vi "Verify Acquisition.vi"(8 "error in (no error)":errorcluster, 11 "CCDCamera in":refnum<class "Real Camera.lvclass">) -> (0 "error out":errorcluster, 3 "CCDCamera out":refnum<class "Real Camera.lvclass">)   [LabVIEW 2018, in "Real Camera.lvclass"]
doc: "Verify acquisition\n\nIf the camera is acquiring, the CCD status will be ACTIVE. Otherwise, it will be IDLE."
uses:
  Real Camera.lvclass
  C:/Users/Denis/Desktop/S4CCS/S4CCS/Simulated_CCD_Camera/Simulated Camera.lvclass
  Simulated_CCD_Camera/Simulated Camera.lvclass
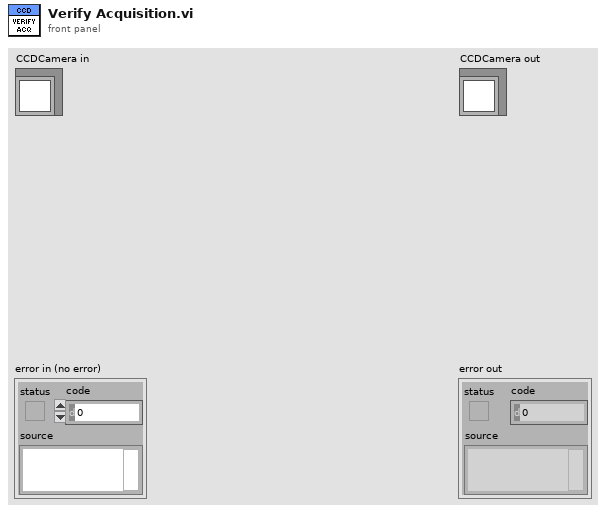
[diagram p1: front panel]
types:
  T1 = typedef "Error Code Enum typedef.ctl" = enum32{"N/A (0)", "DRV_ERROR_CODES", "DRV_SUCCESS", "DRV_VXDNOTINSTALLED", "DRV_ERROR_SCAN", "DRV_ERROR_CHECK_SUM", "DRV_ERROR_FILELOAD", "DRV_UNKNOWN_FUNC", "DRV_ERROR_VXD_INIT", "DRV_ERROR_ADDRESS", "DRV_ERROR_PAGELOCK", "DRV_ERROR_PAGEUNLOCK", "DRV_ERROR_BOARDTEST", "DRV_ERROR_ACK", "DRV_ERROR_UP_FIFO", "DRV_ERROR_PATTERN", "N/A (16)", "DRV_ACQUISITION_ERRORS", "DRV_ACQ_BUFFER", "DRV_ACQ_DOWNFIFO_FULL", "DRV_PROC_UNKONWN_INSTRUCTION", "DRV_ILLEGAL_OP_CODE", "DRV_KINETIC_TIME_NOT_MET", "DRV_ACCUM_TIME_NOT_MET", "DRV_NO_NEW_DATA", "N/A (25)", "DRV_SPOOLERROR", "N/A (27)", "N/A (28)", "N/A (29)", "N/A (30)", "N/A (31)", "N/A (32)", "DRV_TEMPERATURE_CODES", "DRV_TEMPERATURE_OFF", "DRV_TEMPERATURE_NOT_STABILIZED", "DRV_TEMPERATURE_STABILIZED", "DRV_TEMPERATURE_NOT_REACHED", "DRV_TEMPERATURE_OUT_RANGE", "DRV_TEMPERATURE_NOT_SUPPORTED", "DRV_TEMPERATURE_DRIFT", "N/A (41)", "N/A (42)", "N/A (43)", "N/A (44)", "N/A (45)", "N/A (46)", "N/A (47)", "N/A (48)", "DRV_GENERAL_ERRORS", "DRV_INVALID_AUX", "DRV_COF_NOTLOADED", "DRV_FPGAPROG", "DRV_FLEXERROR", "DRV_GPIBERROR", "N/A (55)", "N/A (56)", "N/A (57)", "N/A (58)", "N/A (59)", "N/A (60)", "N/A (61)", "N/A (62)", "N/A (63)", "DRV_DATATYPE", "DRV_DRIVER_ERRORS", "DRV_P1INVALID", "DRV_P2INVALID", "DRV_P3INVALID", "DRV_P4INVALID", "DRV_INIERROR", "DRV_COFERROR", "DRV_ACQUIRING", "DRV_IDLE", "DRV_TEMPCYCLE", "DRV_NOT_INITIALIZED", "DRV_P5INVALID", "DRV_P6INVALID", "DRV_INVALID_MODE", "DRV_INVALID_FILTER", "DRV_I2CERRORS", "DRV_I2CDEVNOTFOUND", "DRV_I2CTIMEOUT", "DRV_P7INVALID", "N/A (84)", "N/A (85)", "N/A (86)", "N/A (87)", "N/A (88)", "N/A (89)", "DRV_IOCERROR", "DRV_VRMVERSIONERROR"}
  T2 = cluster{"CYCLES_DONE":u16, "LAST_IMAGE_NAME":string, "USED_DISK_SPACE":u16, "FRAMES_DONE":u16, "CCD_STATUS":string, "CURRENT_TEMPERATURE":i16, "TEMPERATURE_STATUS":string, "FRAME_EXPOSURE_TIME":sgl, "ERROR":bool, "SERIAL_NUMBER":u16, "ACQUIRING":bool, "IMAGE_INDEX":u32, "SEQS_DONE":u16}
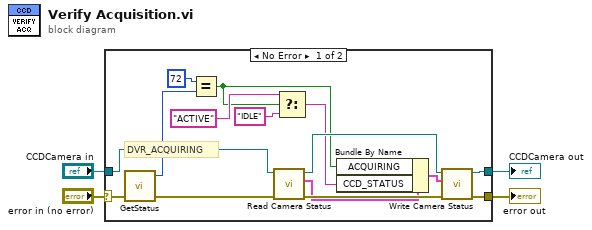
[diagram p0: block diagram]
diagram:
  n1 = case shown="No Error" "error in (no error)" {
    selector: "error in (no error)" -> [w19 w21]
    tunnel: [w16 w21] -> w3
    tunnel: [w15 w20] -> w1
    tunnel: "CCDCamera in" -> [w14 w20]
    frame No Error {
      # "DVR_ACQUIRING"
      n2 = call <userlib>:"GetStatus.vi"("error in (no error)"=w19) -> ("error out"=w11:errorcluster, "status"=w17:T1)  [unwired: 2 in, 1 out]
      n3 = Equal?(x=72, y=w17) -> (x = y?=w7:bool)
      n4 = call "Read Camera Status.vi"("error in (no error)"=w11, "CCDCamera in"=w14) -> ("error out"=w12:errorcluster, "Camera Status"=w9:T2, "CCDCamera out"=w13:refnum<class "Real Camera.lvclass">)  [unwired: 7 in]
      n5 = Select(t="ACTIVE", s=w7, f="IDLE") -> (s? t:f=w6:string)
      n6 = Bundle By Name(cluster=w9, "ACQUIRING"=w7, "CCD_STATUS"=w6) -> (w10:T2)
      n7 = call "Write Camera Status.vi"("error in (no error)"=w12, "Camera Status"=w10, "CCDCamera in"=w13) -> ("error out"=w16:errorcluster, "CCDCamera out"=w15:refnum<class "Real Camera.lvclass">)  [unwired: 7 in]
    }
    frame Error {
    }
  }
  "error out" <- w3
  "CCDCamera out" <- w1
